vi "FindColumnName.vi"(0 "Sequence Context":T1, 5 "start cell in":cluster{"row":i32, "column":i32}, 9 "Column Name":string, 11 "error in (no error)":errorcluster) -> (6 "start cell out":cluster{"row":i32, "column":i32}, 15 "error out":errorcluster)   [LabVIEW 2015]
doc: "This vi will search the array of column headers to find the index of the disired column\nit will then put that number in the start cell out cluster"
uses:
  <vilib>/addons/TestStand/_TSLegacy.llb/LabVIEW Test - Sequence Context.ctl
  <vilib>/addons/TestStand/_TSUtility.llb/TestStand - Get Property Value (String Array).vi
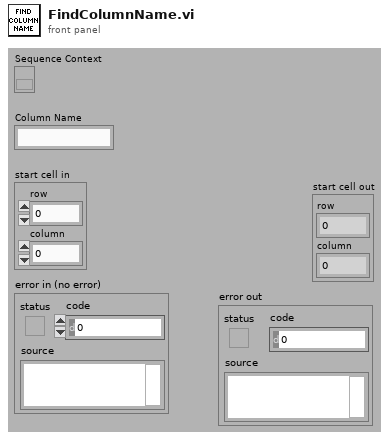
[diagram p1: front panel]
types:
  T1 = typedef "LabVIEW Test - Sequence Context.ctl" = refnum<k7>
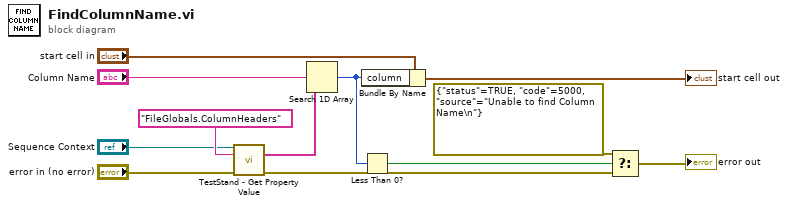
[diagram p0: block diagram]
diagram:
  n1 = call-poly <vilib>:"TestStand - Get Property Value.vi"("Sequence Context In"="Sequence Context", "Lookup String"="FileGlobals.ColumnHeaders", "error in (no error)"="error in (no error)") -> ("Value"=w7:string[], "error out"=w5:errorcluster)  [unwired: 10 in, 1 out]
  n2 = Search 1D Array(1D array=w7, element="Column Name") -> (index of element=w6:i32)  [unwired: 1 in]
  n3 = Bundle By Name(cluster="start cell in", "column"=w6) -> (→"start cell out":cluster{"row":i32, "column":i32})
  n4 = Less Than 0?(x=w6) -> (x < 0?=w1:bool)
  n5 = Select(t=errorcluster {"status"=TRUE, "code"=5000, "source"="Unable to find Column Name\n"}, s=w1, f=w5) -> (s? t:f=→"error out":errorcluster)
